vi "data insert.vi"(8 "error in (no error)":errorcluster, 10 "data in":T1, 11 "table":string) -> (0 "error out":errorcluster)   [LabVIEW 2016, in "采配水.lvlib"]
uses:
  <vilib>/addons/database/Auxilliary.llb/DB Tools Column Info.ctl
  <vilib>/addons/database/Auxilliary.llb/DB Tools DataTypes.ctl
  <vilib>/addons/database/NI_Database_API.lvlib
  AIRMAR WeatherCaster/AIRMAR WeatherCaster.lvlib
  <vilib>/Utility/VariantDataType/VariantType.lvlib
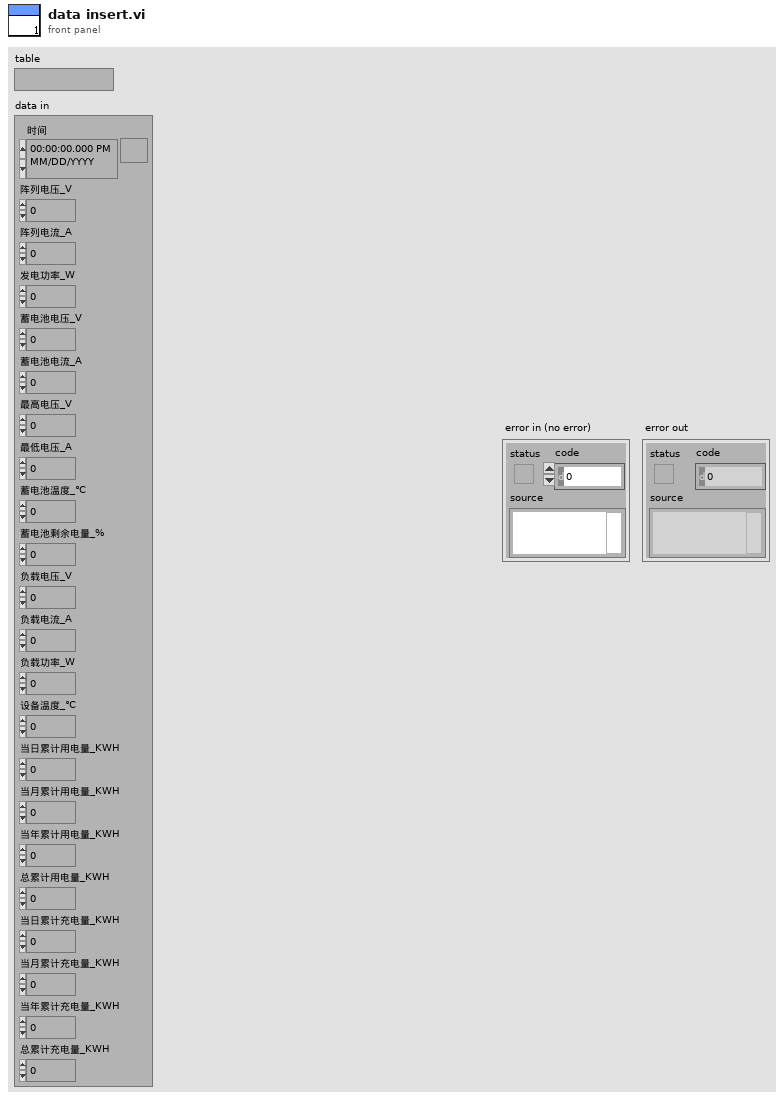
[diagram p1: front panel]
types:
  T1 = cluster{"时间":timestamp, "阵列电压_V":dbl, "阵列电流_A":dbl, "发电功率_W":dbl, "蓄电池电压_V":dbl, "蓄电池电流_A":dbl, "最高电压_V":dbl, "最低电压_A":dbl, "蓄电池温度_℃":dbl, "蓄电池剩余电量_%":dbl, "负载电压_V":dbl, "负载电流_A":dbl, "负载功率_W":dbl, "设备温度_℃":dbl, "当日累计用电量_KWH":dbl, "当月累计用电量_KWH":dbl, "当年累计用电量_KWH":dbl, "总累计用电量_KWH":dbl, "当日累计充电量_KWH":dbl, "当月累计充电量_KWH":dbl, "当年累计充电量_KWH":dbl, "总累计充电量_KWH":dbl}
  T2 = typedef "NI_Database_API.lvlib/DB Tools Column Info.ctl" = cluster{"column name":string, "data type":T3, "size":i32, "allow null?":bool}
  T3 = typedef "NI_Database_API.lvlib/DB Tools DataTypes.ctl" = enum16{"String", "Long (I32)", "Single (SGL)", "Double (DBL)", "Date/Time", "Binary"}
  T4 = typedef "VariantType.lvlib/Type.ctl" = enum8{"Invalid Type", "Void", "I8", "I16", "I32", "I64", "U8", "U16", "U32", "U64", "Single Float", "Double Float", "Extended Float", "Single Complex", "Double Complex", "Extended Complex", "Enum U8", "Enum U16", "Enum U32", "Enum U64", "Single Float With Unit", "Double Float With Unit", "Extended Float With Unit", "Single Complex with Unit", "Double Complex with Unit", "Extended Complex with Unit", "Boolean", "String", "Path", "Picture", "Tag", "Array", "Cluster", "Variant", "LV Variant", "Waveform", "Timestamp", "Digital Waveform", "Digital Data", "ExpressData", "Refnum", "External Data", "VI", "Poly VI", "LabVIEW Class Instance", "Fixed Point"}
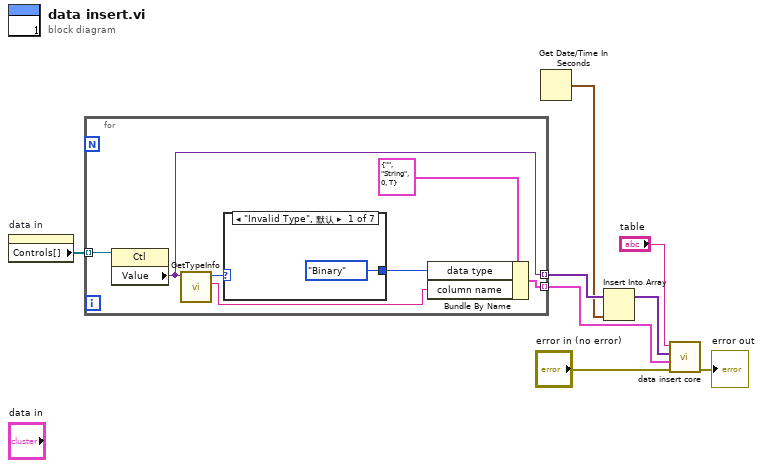
[diagram p0: block diagram]
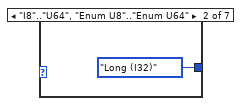
[diagram p2: hidden frame]
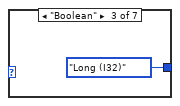
[diagram p3: hidden frame]
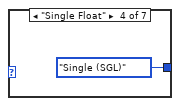
[diagram p4: hidden frame]
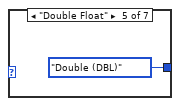
[diagram p5: hidden frame]
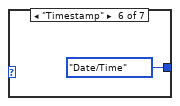
[diagram p6: hidden frame]
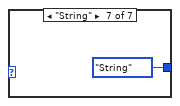
[diagram p7: hidden frame]
diagram:
  n1 = property on="data in" class="Clust (严格)"() -> ("Controls[]"=w8:refnum<vi>[])  [unwired: 2 in, 2 out]
  n2 = for {
    tunnel: w8 -> [w15] mode=indexing
    tunnel: [w9] -> w7 mode=indexing
    tunnel: [w10] -> w2 mode=indexing
    n3 = property class="Ctl"(reference=w15) -> ("Value"=w9:variant)  [unwired: 1 in, 2 out]
    n4 = call <vilib>:"GetTypeInfo.vi"("Variant"=w9) -> ("Name"=w13:string, "Type Enum"=w12:T4)  [unwired: 6 in, 3 out]
    n5 = case shown="\"Invalid Type\", 默认" w12 {
      tunnel: [DB_Tools_DataTypes."Binary" ("data type") DB_Tools_DataTypes."Long (I32)" ("data type") DB_Tools_DataTypes."Long (I32)" ("data type") DB_Tools_DataTypes."Single (SGL)" ("data type") DB_Tools_DataTypes."Double (DBL)" ("data type") DB_Tools_DataTypes."Date/Time" ("data type") DB_Tools_DataTypes."String" ("data type")] -> w11
      frame "Invalid Type", Default {
      }
      frame "I8".."U64", "Enum U8".."Enum U64" {
      }
      frame "Boolean" {
      }
      frame "Single Float" {
      }
      frame "Double Float" {
      }
      frame "Timestamp" {
      }
      frame "String" {
      }
    }
    n6 = Bundle By Name(cluster=T2 {"column name"="", "data type"=enum."String", "size"=0, "allow null?"=TRUE} ("column information"), "data type"=w11, "column name"=w13) -> (w10:T2)
  }
  n7 = Get Date/Time In Seconds() -> (seconds since 1Jan1904=w6:timestamp)
  n8 = Insert Into Array(array=w7, new element=w6) -> (w5:variant[])  [unwired: 1 in]
  n9 = call "data insert core.vi"("error in (no error)"="error in (no error)", "column information"=w2, "data"=w5, "table"="table") -> ("error out"=→"error out":errorcluster)  [unwired: 7 in]
